vi "Get Resource Type.vi"(4 "GPIO in":refnum<class "GPIO.lvclass">) -> (7 "Resource Type":string)   [LabVIEW 2024, in "CTI.lvlib" / "GPIO.lvclass"]
uses:
  GPIO.lvclass
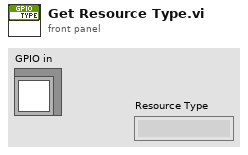
[diagram p1: front panel]
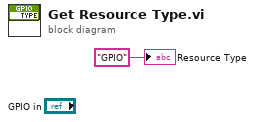
[diagram p0: block diagram]
diagram:
  "Resource Type" <- "GPIO" ("Resource Type")
